vi "UART Read Bytes.vi"(7 "pLen":u16, 9 "UARTIndex":i32, 10 "DevIndex":i32, 11 "DevType":i32) -> (2 "function return":i32, 3 "pReadData":u8[](array[numeric]), 5 "pLen out":u16)   [LabVIEW 2010, in "ControlUART.lvlib"]
doc: "int WINAPI UART_ReadBytes(int DevType,int DevIndex,int UARTIndex,unsigned char *pReadData,unsigned short *pLen);"
uses:
  ControlUART.lvlib
  ControlUART/Ginkgo_Driver.dll
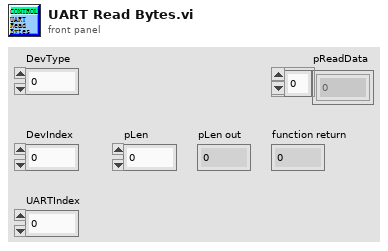
[diagram p1: front panel]
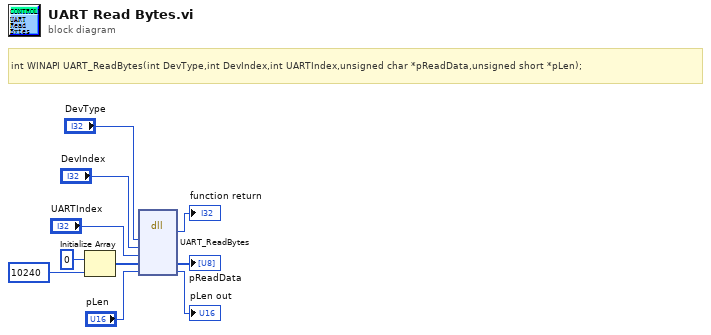
[diagram p0: block diagram]
diagram:
  # "int WINAPI UART_ReadBytes(int DevType,int DevIndex,int UARTIndex,unsigned char *pReadData,unsigned short *pLen);"
  n1 = Initialize Array(u8 0 ("element"), 10240 ("dimension size")) -> (w6:u8[])
  n2 = dll-call lib="E:/Project/vt_ginkgo/truck/Ginkgo Driver/vs2010/Ginkgo_USB-I2C&SPI&CAN_API_v2.0.3.3/lib/labview_32bit/ControlUART/Ginkgo_Driver.*" fn="UART_ReadBytes"("DevType"="DevType", "DevIndex"="DevIndex", "UARTIndex"="UARTIndex", "pReadData"=w6, "pLen"="pLen") -> (→"function return":i32, "pReadData"=→"pReadData":u8[], "pLen"=→"pLen out":u16)  [unwired: 6 in, 2 out]
